vi "XAINSCFG.VI"(0 "BoardNum":i32, 5 "LowChan":i32, 7 "HighChan":i32, 9 "Count":i32=1000, 11 "Rate":i32=1000, 12 "Range":i32(ring)=2 items=["Not Programmable"=0, "+- 20 V"=27, "+- 10 V"=1, "+- 5 V"=2, "+- 4 V"=28, "+- 2.5 V"=3, "+- 2 V"=29, "+- 1.67 V"=4, "+- 1.25 V"=5, "+- 1 V"=6, "+- .625 V"=7, "+- .5 V"=8, "+- .25 V"=30, "+- .2 V"=31, "+- .1 V"=9, "+- .05 V"=10, "+- .01 V"=11, "+- .005 V"=12, "0 - 10 V"=13, "0 - 5 V"=14, "0 - 4 V"=36, "0 - 2.5 V"=15, "0 - 2 V"=16, "0 - 1.67 V"=17, "0 - 1.25 V"=18, "0 - 1 V"=19, "0 - .5 V"=32, "0 - .25 V"=33, "0 - .2 V"=34, "0 - .1 V"=20, "0 - .02 V"=35, "0 - .01 V"=21, "4 - 20 mA"=22, "2 - 10 mA"=23, "1 - 5 mA"=24, ".5 - 2.5 mA"=25, "0 - 20 mA"=26], 13 "InterChannel Delay":dbl=-1.0 format="%.2f") -> (1 "ActualRate":i32, 3 "ErrMsg":string, 4 "Voltage Data Array 2":sgl[](array[numeric])=[0.011444092, 0.011444092, 0.010681152, 0.011291504, 0.011291504, 0.011444092, 0.011291504, 0.010223389, 0.010223389, 0.010070801, 0.010681152, 0.011291504, 0.010070801, 0.010223389, 0.009918213, 0.010070801, 0.009765625, 0.009765625, 0.010070801, 0.009307861, 0.009460449, 0.009155273, 0.009765625, 0.009155273, 0.009460449, 0.009460449, 0.009307861, 0.010070801, 0.009918213, 0.00869751, 0.008392334, 0.00869751, 0.009155273, 0.009002686, 0.008392334, 0.008850098, 0.008392334, 0.008850098, 0.008392334, 0.009155273, 0.008392334, 0.00869751, 0.008850098, 0.0076293945, 0.009307861, 0.008087158, 0.00793457, 0.0077819824, 0.008392334, 0.008087158, 0.0076293945, 0.008392334, 0.008239746, 0.0073242188, 0.0077819824, 0.0076293945, 0.008239746, 0.0074768066, 0.0073242188, 0.008392334, 0.007171631, 0.0074768066, 0.0076293945, 0.0076293945, 0.006713867, 0.0076293945, 0.0064086914, 0.007171631, 0.0074768066, 0.0076293945, 0.007171631, 0.0076293945, 0.007019043, 0.0073242188, 0.007019043, 0.0065612793, 0.006713867, 0.006866455, 0.0076293945, 0.0073242188, 0.0065612793, 0.0073242188, 0.0062561035, 0.0076293945, 0.007019043, 0.0065612793, 0.007019043, 0.006866455, 0.0065612793, 0.006713867, 0.006713867, 0.0062561035, 0.0065612793, 0.0062561035, 0.006713867, 0.006713867, 0.0065612793, 0.005645752, 0.006866455, 0.0064086914, 0.006713867, 0.0065612793, 0.0064086914, 0.0065612793, 0.007019043, 0.007171631, 0.0076293945, 0.007019043, 0.0074768066, 0.006866455, 0.007019043, 0.007171631, 0.007019043, 0.008239746, 0.008392334, 0.008239746, 0.008544922, 0.008544922, 0.009002686, 0.010986328, 0.01159668, 0.0132751465, 0.015563965, 0.018157959, 0.023040771, 0.030822754, 0.04257202, 0.057678223, 0.066986084, 0.06072998, 0.044708252, 0.03173828, 0.023651123, 0.018310547, 0.014801025, 0.012512207, 0.011138916, 0.009765625, 0.008544922, 0.008087158, 0.00793457, 0.00793457, 0.007171631, 0.007171631, 0.006713867, 0.0059509277, 0.0062561035, 0.006866455, 0.006866455, 0.007019043, 0.0064086914, 0.0061035156, 0.006866455, 0.007019043, 0.0064086914, 0.006866455, 0.0064086914, 0.0064086914, 0.0065612793, 0.0061035156, 0.0061035156, 0.0061035156, 0.0062561035, 0.005645752, 0.0061035156, 0.0059509277, 0.0062561035, 0.0061035156, 0.0062561035, 0.005493164, 0.0059509277, 0.00579834, 0.0065612793, 0.005493164, 0.0059509277, 0.0059509277, 0.0062561035, 0.0065612793, 0.0059509277, 0.0062561035, 0.00579834, 0.006866455, 0.0065612793, 0.0059509277, 0.00579834, 0.00579834, 0.0065612793, 0.007171631, 0.0064086914, 0.006866455, 0.007019043, 0.0073242188, 0.0064086914, 0.006713867, 0.0062561035, 0.006866455, 0.007171631, 0.0073242188, 0.0065612793, 0.007019043, 0.006713867, 0.0065612793, 0.006866455, 0.006713867, 0.0073242188, 0.006713867, 0.0074768066, 0.006866455, 0.0076293945, 0.0065612793, 0.0077819824, 0.0077819824, 0.007019043, 0.008239746, 0.0073242188, 0.0074768066, 0.0077819824, 0.0076293945, 0.0076293945, 0.008239746, 0.008087158, 0.0076293945, 0.00793457, 0.0077819824, 0.00793457, 0.00793457, 0.0073242188, 0.00793457, 0.008544922, 0.0076293945, 0.008544922, 0.008850098, 0.008239746, 0.008544922, 0.008544922, 0.008239746, 0.009460449, 0.008850098, 0.009307861, 0.008850098, 0.009765625, 0.009002686, 0.008544922, 0.00869751, 0.009002686, 0.00869751, 0.008850098, 0.009765625, 0.009460449, 0.009460449, 0.009460449] format="%.4f", 15 "Data Array":sgl[][](array[numeric]) format="%.4f")   [LabVIEW 2013]
uses:
  Das16.llb/ToEng(array).vi
panel:
  out "?":sgl[][](graph)
  in  "Mode":i32(ring) items=["DEFAULTIO", "SINGLEIO", "DMAIO", "BLOCKIO", "BURSTIO"]
  in  "ExtMemory":bool
  in  "DTConnect":bool
  in  "ConvertData":bool
  in  "Extclock":bool
  # "AInScFg.VI Inputs:"
  # "Demo for the function cbAInScan(). \n\nMultiple analog input, foreground operation."
  # "Channel Index"
  # "Sample No."
  # "Results:"
  # "Options parameters (input to OptAIn.VI).\nDefault used for other option parameters."
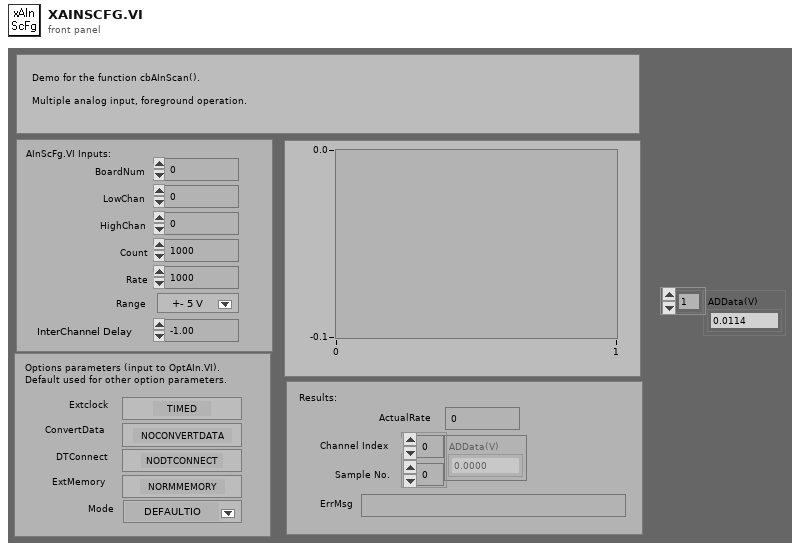
[diagram p1: front panel]
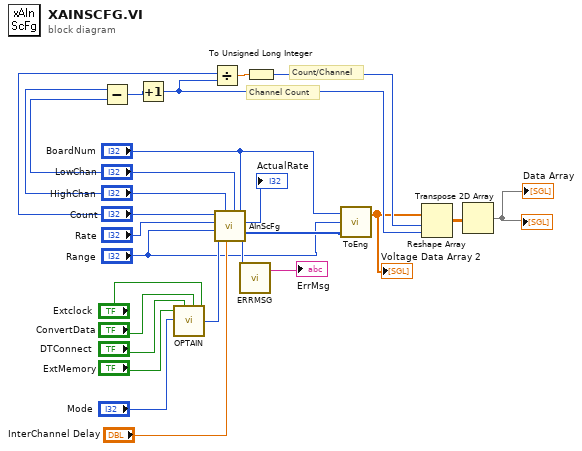
[diagram p0: block diagram]
diagram:
  # "Count/Channel"
  # "Channel Count"
  n1 = Subtract(x="HighChan", y="LowChan") -> (x-y=w8:i32)
  n2 = Increment(x=w8) -> (x+1=w4:i32)
  n3 = call "OPTAIN.VI"("ExtMemory(false)"="ExtMemory", "DTConnect(false)"="DTConnect", "Mode"="Mode", "ConvertData(false)"="ConvertData", "Extclock(false)"="Extclock") -> ("AInScanOptions"=w15:u32)  [unwired: 4 in]
  n4 = Divide(x="Count", y=w4) -> (x/y=w10:dbl)
  n5 = call "AInScFg.VI"("BoardNum"="BoardNum", "LowChan"="LowChan", "InterChannel Delay"="InterChannel Delay", "HighChan"="HighChan", "Options"=w15, "Range"="Range", "Rate"="Rate", "Count"="Count") -> ("ErrCode"=w14:i32, "ADData"=w7:u16[], "Rate"=→"ActualRate":i32)
  n6 = call "ERRMSG.VI"("ErrCode"=w14) -> ("ErrMsg"=→"ErrMsg":string)  [unwired: 1 out]
  n7 = To Unsigned Long Integer(number=w10) -> (unsigned 32bit integer=w9:u32)
  n8 = call-poly "ToEng.VI"("AD Data"=w7, "Range"="Range", "BoardNum"="BoardNum") -> ("Eng Units"=w1:sgl[])  [unwired: 1 out]
  "Voltage Data Array 2" <- w1
  n9 = Reshape Array(w1, w9, w4) -> (w3:sgl[][])
  n10 = Transpose 2D Array(2D array=w3) -> (transposed array=→"?" →"Data Array":sgl[][])
